vi "RT_Act_Plant_5ms_2_v1 (SubVI).vi"(9 "not.Sim_Running":bool, 11 "TVA_cmd":dbl[](array[numeric])) -> (0 "Act_b i-2":dbl[](array[numeric]), 1 "Act_b i-1":dbl[](array[numeric]), 3 "Act_b":dbl[](array[numeric]))   [LabVIEW 2017]
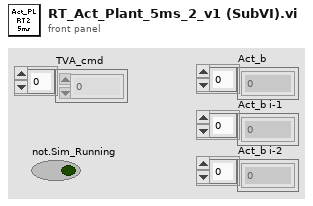
[diagram p1: front panel]
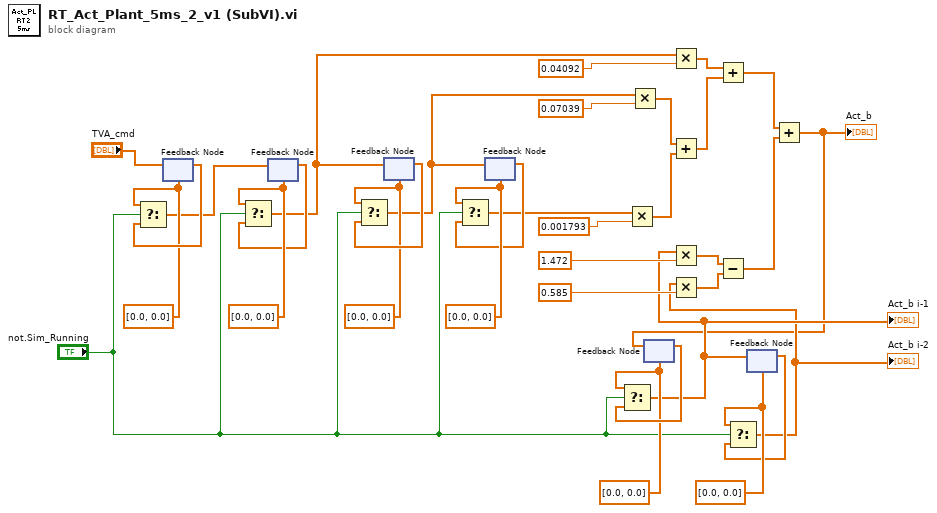
[diagram p0: block diagram]
diagram:
  w10 = dbl[] [0.0, 0.0] ("TVA_cmd")
  w12 = dbl[] [0.0, 0.0] ("TVA_cmd")
  w15 = dbl[] [0.0, 0.0] ("TVA_cmd")
  w17 = dbl[] [0.0, 0.0] ("TVA_cmd")
  w20 = dbl[] [0.0, 0.0] ("TVA_cmd")
  w18 = dbl[] [0.0, 0.0] ("TVA_b")
  n1 = feedback #1(w20) -> (w21:dbl[])
  n2 = Select(t=w20, s="not.Sim_Running", f=w21) -> (s? t:f=w11:dbl[])
  n3 = feedback-in #1("TVA_cmd") -> ()
  n4 = feedback #2(w15) -> (w14:dbl[])
  n5 = Select(t=w15, s="not.Sim_Running", f=w14) -> (s? t:f=w3:dbl[])
  n6 = feedback-in #2(w11) -> ()
  n7 = feedback #3(w12) -> (w13:dbl[])
  n8 = Select(t=w12, s="not.Sim_Running", f=w13) -> (s? t:f=w4:dbl[])
  n9 = feedback-in #3(w3) -> ()
  n10 = feedback #4(w10) -> (w9:dbl[])
  n11 = Select(t=w10, s="not.Sim_Running", f=w9) -> (s? t:f=w5:dbl[])
  n12 = feedback-in #4(w4) -> ()
  n13 = Multiply(x=w5, y=0.001793) -> (x*y=w27:dbl[])
  n14 = Multiply(x=w4, y=0.07039) -> (x*y=w28:dbl[])
  n15 = feedback #5(w18) -> (w19:dbl[])
  n16 = Select(t=w18, s="not.Sim_Running", f=w19) -> (s? t:f=w8:dbl[])
  "Act_b i-1" <- w8
  n17 = Multiply(x=w3, y=0.04092) -> (x*y=w24:dbl[])
  n18 = Add(x=w28, y=w27) -> (x+y=w23:dbl[])
  n19 = Multiply(x=w8, y=1.472) -> (x*y=w32:dbl[])
  n20 = Add(x=w24, y=w23) -> (x+y=w22:dbl[])
  n21 = feedback #6(w17) -> (w16:dbl[])
  n22 = Select(t=w17, s="not.Sim_Running", f=w16) -> (s? t:f=w7:dbl[])
  "Act_b i-2" <- w7
  n23 = Multiply(x=w7, y=0.585) -> (x*y=w31:dbl[])
  n24 = Subtract(x=w32, y=w31) -> (x-y=w26:dbl[])
  n25 = feedback-in #6(w8) -> ()
  n26 = Add(x=w22, y=w26) -> (x+y=w6:dbl[])
  "Act_b" <- w6
  n27 = feedback-in #5(w6) -> ()
